vi "Double Solenoid Control.vi"   [LabVIEW 2015]
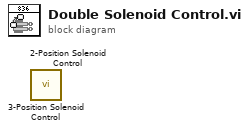
[diagram p0: block diagram]
diagram:
  n1 = call <userlib>:"3-Position Solenoid Control.vi"() -> ()  [unwired: 9 in, 3 out]
  n2 = call <userlib>:"2-Position Solenoid Control.vi"() -> ()  [unwired: 9 in, 3 out]
